vi "Variable@LRemove__Parameter.vi"(1 "ParamterIn":string) -> (0 "ParamterOut":string)   [LabVIEW 2019]
panel:
  in  "Section":string(combo)
  in  "Value":string(combo)
  in  "ParameterName":string(combo)
  in  "Confirm":bool
  # "Variable@LRemove $Variable,$Value(,$Section)"
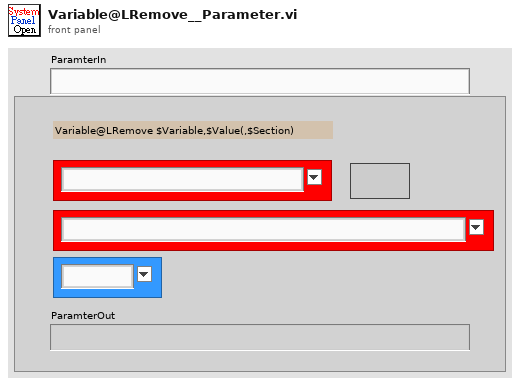
[diagram p1: front panel]
types:
  T1 = enum16{"Get", "Init", "Set", "Delete", "GetElement", "Inc", "Dec", "ReName"}
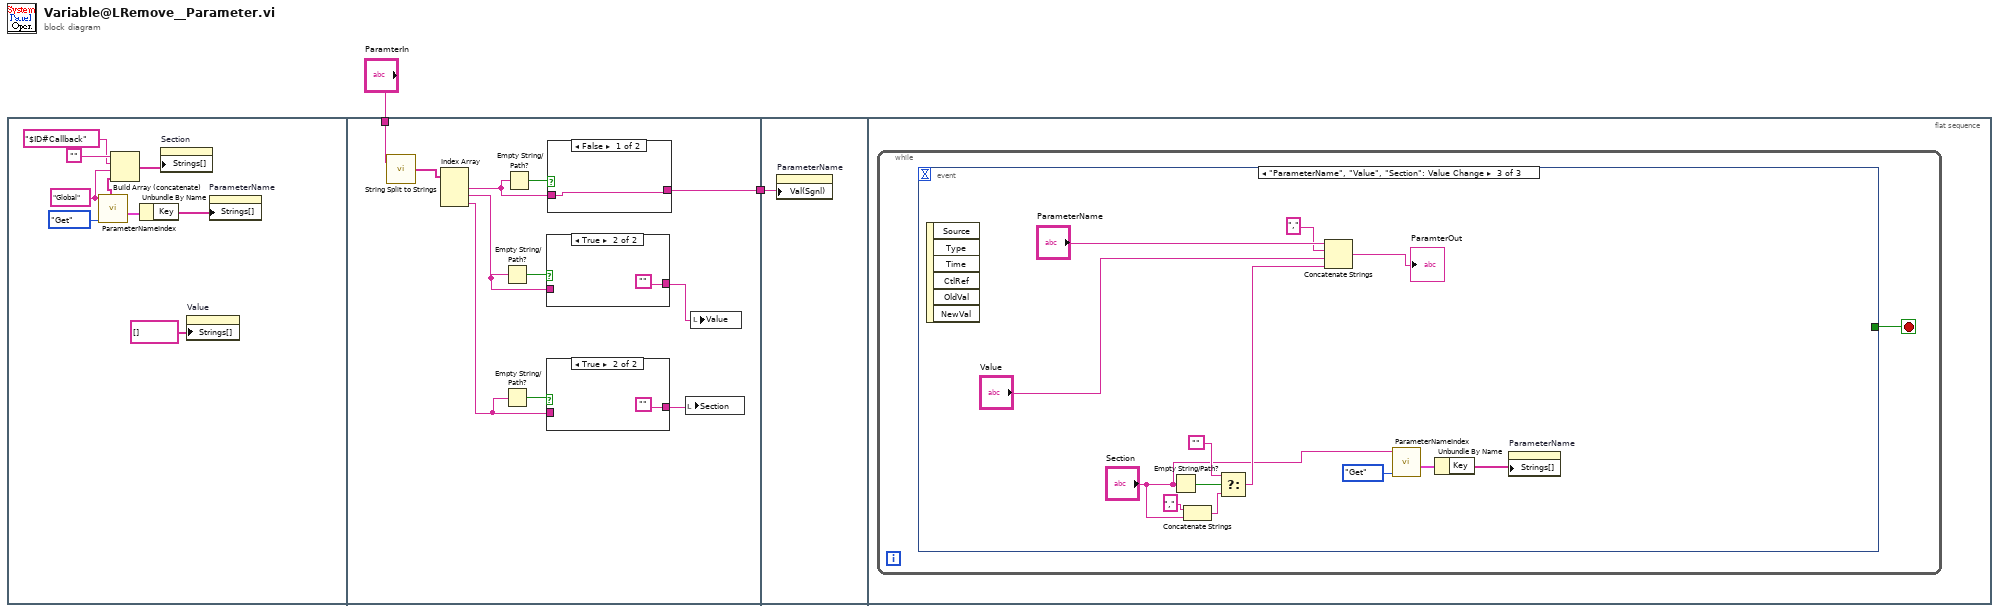
[diagram p0: block diagram]
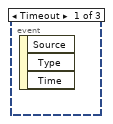
[diagram p5: hidden frame]
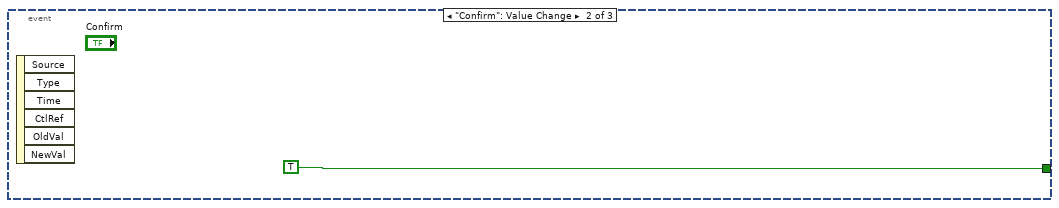
[diagram p6: hidden frame]
diagram:
  n1 = flat-sequence {
    tunnel: "ParamterIn" -> [w18]
    tunnel: [w20] -> w1
    tunnel: w1 -> [w29]
    frame #0 {
      w5 = "Global" ("VariableSection")
      n2 = call "ParameterNameIndex.vi"("OP"=T1."Get", "VariableSection"=w5) -> ("GlobalKeyValue"=w11:cluster{"Key":string[], "Value":string[]}, "SectionList"=w6:string[])  [unwired: 3 in, 5 out]
      n3 = Build Array (concatenate)("", "$ID#Callback" ("VariableSection"), w5, w6) -> (w4:string[])
      n4 = Unbundle By Name(w11) -> ("Key"=w10:string[])
      n5 = property on="Section" class="CmbBox"("Strings[]"=w4) -> ()  [unwired: 2 in, 2 out]
      n6 = property on="Value" class="CmbBox"("Strings[]"=string[] [] ("Strings []")) -> ()  [unwired: 2 in, 2 out]
      n7 = property on="ParameterName" class="CmbBox"("Strings[]"=w10) -> ()  [unwired: 2 in, 2 out]
    }
    frame #1 {
      n8 = call "String Split to Strings.vi"("String"=w18) -> ("Array"=w17:string[])  [unwired: 1 in]
      n9 = Index Array(array=w17) -> (element #1=w16:string, element #2=w15:string, element #3=w13:string)  [unwired: 3 in]
      n10 = Empty String/Path?(string/path=w15) -> (empty?=w21:bool)
      n11 = Empty String/Path?(string/path=w13) -> (empty?=w14:bool)
      n12 = Empty String/Path?(string/path=w16) -> (empty?=w22:bool)
      n13 = case shown="True" w21 {
        tunnel: w15 -> [w25 _]
        tunnel: [w25 ""] -> w19
        frame False {
        }
        frame True {
        }
      }
      n14 = case shown="True" w14 {
        tunnel: w13 -> [w23 _]
        tunnel: [w23 ""] -> w12
        frame False {
        }
        frame True {
        }
      }
      n15 = case shown="False" w22 {
        tunnel: w16 -> [w27 w28]
        tunnel: [w27 w28] -> w20
        frame False {
        }
        frame True {
        }
      }
      n16 = local write "Section"(w12) -> ()
      n17 = local write "Value"(w19) -> ()
    }
    frame #2 {
      n18 = property on="ParameterName" class="CmbBox"("Val(Sgnl)"=w29) -> ()  [unwired: 2 in, 2 out]
    }
    frame #3 {
      n19 = while {
        stop <- w30 stop-if-true
        n20 = event shown="[2] \"ParameterName\", \"Value\", \"Section\": Value Change" {
          selector: _ -> [_ _ _]
          dyn-events: _ -> [_ _ _]
          timeout: _ -> [_ _ _]
          tunnel: [_ TRUE _] -> w30
          event Timeout {
            n21 = event-data() -> ()  [unwired: 1 in, 3 out]
          }
          event "Confirm": Value Change {
            n22 = event-data() -> ()  [unwired: 1 in, 6 out]
          }
          event "ParameterName", "Value", "Section": Value Change {
            n23 = event-data() -> ()  [unwired: 1 in, 6 out]
            n24 = Empty String/Path?(string/path="Section") -> (empty?=w40:bool)
            n25 = Concatenate Strings("," ("string"), "Section") -> (w41:string)
            n26 = Select(t="", s=w40, f=w41) -> (s? t:f=w38:string)
            n27 = Concatenate Strings("ParameterName", "," ("string"), "Value", w38) -> (→"ParamterOut":string)
            n28 = call "ParameterNameIndex.vi"("OP"=T1."Get", "VariableSection"="Section") -> ("GlobalKeyValue"=w33:cluster{"Key":string[], "Value":string[]})  [unwired: 3 in, 6 out]
            n29 = Unbundle By Name(w33) -> ("Key"=w39:string[])
            n30 = property on="ParameterName" class="CmbBox"("Strings[]"=w39) -> ()  [unwired: 2 in, 2 out]
          }
        }
      }
    }
  }
